vi "Temperhum.Open.vi"(8 "error in (no error)":errorcluster) -> (0 "error out":errorcluster, 2 "Computer Name":string, 3 "Device Handle":i64)   [LabVIEW 2019, in "TEMPerHUM.lvlib"]
uses:
  TEMPerHUM.lvlib
  RDingUSB.dll
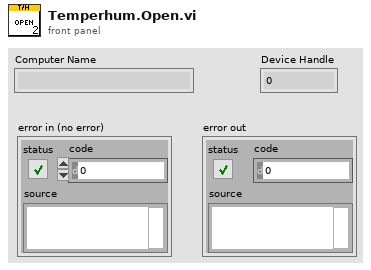
[diagram p1: front panel]
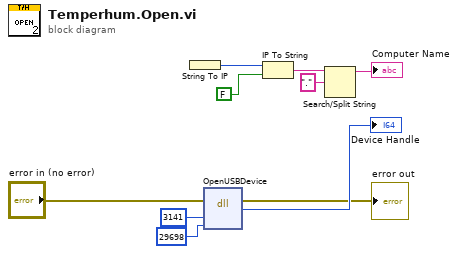
[diagram p0: block diagram]
diagram:
  n1 = String To IP() -> (0:w5:u32)  [unwired: 1 in]
  n2 = dll-call lib="C:/Users/Ranjani/Documents/GitHub/Temperhum-Instrument/lvsrc/SMOs/TEMPerHUM/RDingUSB.dll" fn="OpenUSBDevice"(error in="error in (no error)", "VID"=3141, "PID"=29698) -> (error out=→"error out":errorcluster, "return type"=→"Device Handle":i64)  [unwired: 4 in, 1 out]
  n3 = IP To String(1:FALSE, 2:w5) -> (0:w1:string)
  n4 = Search/Split String(string=w1, search string/char (-)=".") -> (substring before match=→"Computer Name":string)  [unwired: 1 in, 2 out]
